vi "multi-function-fpga3.vi"() -> ()   [LabVIEW 2016]
uses:
  <vilib>/rvi/Emulation/niFpgaGetClockAttributes.vi
  <vilib>/rvi/Emulation/niFpgaSctlEmulationGetInTimedLoop.vi
  <vilib>/rvi/Emulation/niFpgaEmulationReportErrorSimple.vi
  <vilib>/rvi/eio/common/nirviEmuTemplateMethod_errors.vi
  <vilib>/rvi/Emulation/niFpgaCriticalErrorInLSC.vi
  <vilib>/eio/EIONode/EIONode.xnode
panel:
  in  "Reset buttons":T1
  in  "Channel15":T2={"Ctrl"=enum."OFF", "scan end"=3.5, "scan begin"=0.0, "scan step"=0.0, "main input"=enum."DIO0", "sub input"=enum."DIO0", "boolean low"=3.5, "boolean high"=0.0} {"boolean high" format="%#_17g"; "boolean low" format="%#_17g"; "scan step" format="%#_17g"; "scan begin" format="%#_17g"; "scan end" format="%#_17g"}
  in  "Channel14":T2={"Ctrl"=enum."OFF", "scan end"=3.5, "scan begin"=0.0, "scan step"=0.0, "main input"=enum."DIO0", "sub input"=enum."DIO0", "boolean low"=3.5, "boolean high"=0.0} {"boolean high" format="%#_17g"; "boolean low" format="%#_17g"; "scan step" format="%#_17g"; "scan begin" format="%#_17g"; "scan end" format="%#_17g"}
  in  "Channel13":T2={"Ctrl"=enum."OFF", "scan end"=3.5, "scan begin"=0.0, "scan step"=0.0, "main input"=enum."DIO0", "sub input"=enum."DIO0", "boolean low"=3.5, "boolean high"=0.0} {"boolean high" format="%#_17g"; "boolean low" format="%#_17g"; "scan step" format="%#_17g"; "scan begin" format="%#_17g"; "scan end" format="%#_17g"}
  in  "Channel12":T2={"Ctrl"=enum."OFF", "scan end"=3.5, "scan begin"=0.0, "scan step"=0.0, "main input"=enum."DIO0", "sub input"=enum."DIO0", "boolean low"=3.5, "boolean high"=0.0} {"boolean high" format="%#_17g"; "boolean low" format="%#_17g"; "scan step" format="%#_17g"; "scan begin" format="%#_17g"; "scan end" format="%#_17g"}
  in  "Channel11":T2={"Ctrl"=enum."OFF", "scan end"=3.5, "scan begin"=0.0, "scan step"=0.0, "main input"=enum."DIO0", "sub input"=enum."DIO0", "boolean low"=3.5, "boolean high"=0.0} {"boolean high" format="%#_17g"; "boolean low" format="%#_17g"; "scan step" format="%#_17g"; "scan begin" format="%#_17g"; "scan end" format="%#_17g"}
  in  "Channel10":T2={"Ctrl"=enum."OFF", "scan end"=3.5, "scan begin"=0.0, "scan step"=0.0, "main input"=enum."DIO0", "sub input"=enum."DIO0", "boolean low"=3.5, "boolean high"=0.0} {"boolean high" format="%#_17g"; "boolean low" format="%#_17g"; "scan step" format="%#_17g"; "scan begin" format="%#_17g"; "scan end" format="%#_17g"}
  in  "Channel9":T2={"Ctrl"=enum."OFF", "scan end"=3.5, "scan begin"=0.0, "scan step"=0.0, "main input"=enum."DIO0", "sub input"=enum."DIO0", "boolean low"=3.5, "boolean high"=0.0} {"boolean high" format="%#_17g"; "boolean low" format="%#_17g"; "scan step" format="%#_17g"; "scan begin" format="%#_17g"; "scan end" format="%#_17g"}
  in  "Channel8":T2={"Ctrl"=enum."OFF", "scan end"=3.5, "scan begin"=0.0, "scan step"=0.0, "main input"=enum."DIO0", "sub input"=enum."DIO0", "boolean low"=3.5, "boolean high"=0.0} {"boolean high" format="%#_17g"; "boolean low" format="%#_17g"; "scan step" format="%#_17g"; "scan begin" format="%#_17g"; "scan end" format="%#_17g"}
  in  "Channel7":T2={"Ctrl"=enum."OFF", "scan end"=3.5, "scan begin"=0.0, "scan step"=0.0, "main input"=enum."DIO0", "sub input"=enum."DIO0", "boolean low"=3.5, "boolean high"=0.0} {"boolean high" format="%#_17g"; "boolean low" format="%#_17g"; "scan step" format="%#_17g"; "scan begin" format="%#_17g"; "scan end" format="%#_17g"}
  in  "Channel6":T2={"Ctrl"=enum."OFF", "scan end"=3.5, "scan begin"=0.0, "scan step"=0.0, "main input"=enum."DIO0", "sub input"=enum."DIO0", "boolean low"=3.5, "boolean high"=0.0} {"boolean high" format="%#_17g"; "boolean low" format="%#_17g"; "scan step" format="%#_17g"; "scan begin" format="%#_17g"; "scan end" format="%#_17g"}
  in  "Channel5":T2={"Ctrl"=enum."OFF", "scan end"=3.5, "scan begin"=0.0, "scan step"=0.0, "main input"=enum."DIO0", "sub input"=enum."DIO0", "boolean low"=3.5, "boolean high"=0.0} {"boolean high" format="%#_17g"; "boolean low" format="%#_17g"; "scan step" format="%#_17g"; "scan begin" format="%#_17g"; "scan end" format="%#_17g"}
  in  "Channel4":T2={"Ctrl"=enum."OFF", "scan end"=3.5, "scan begin"=0.0, "scan step"=0.0, "main input"=enum."DIO0", "sub input"=enum."DIO0", "boolean low"=3.5, "boolean high"=0.0} {"boolean high" format="%#_17g"; "boolean low" format="%#_17g"; "scan step" format="%#_17g"; "scan begin" format="%#_17g"; "scan end" format="%#_17g"}
  in  "Channel3":T2={"Ctrl"=enum."OFF", "scan end"=3.5, "scan begin"=0.0, "scan step"=0.0, "main input"=enum."DIO0", "sub input"=enum."DIO0", "boolean low"=3.5, "boolean high"=0.0} {"boolean high" format="%#_17g"; "boolean low" format="%#_17g"; "scan step" format="%#_17g"; "scan begin" format="%#_17g"; "scan end" format="%#_17g"}
  in  "Channel2":T2={"Ctrl"=enum."OFF", "scan end"=3.5, "scan begin"=0.0, "scan step"=0.0, "main input"=enum."DIO0", "sub input"=enum."DIO0", "boolean low"=3.5, "boolean high"=0.0} {"boolean high" format="%#_17g"; "boolean low" format="%#_17g"; "scan step" format="%#_17g"; "scan begin" format="%#_17g"; "scan end" format="%#_17g"}
  in  "Channel1":T2={"Ctrl"=enum."OFF", "scan end"=3.5, "scan begin"=0.0, "scan step"=0.0, "main input"=enum."DIO0", "sub input"=enum."DIO0", "boolean low"=3.5, "boolean high"=0.0} {"boolean high" format="%#_17g"; "boolean low" format="%#_17g"; "scan step" format="%#_17g"; "scan begin" format="%#_17g"; "scan end" format="%#_17g"}
  in  "Channel0":T2={"Ctrl"=enum."OFF", "scan end"=3.5, "scan begin"=0.0, "scan step"=0.0, "main input"=enum."DIO0", "sub input"=enum."DIO0", "boolean low"=3.5, "boolean high"=0.0} {"boolean high" format="%#_17g"; "boolean low" format="%#_17g"; "scan step" format="%#_17g"; "scan begin" format="%#_17g"; "scan end" format="%#_17g"}
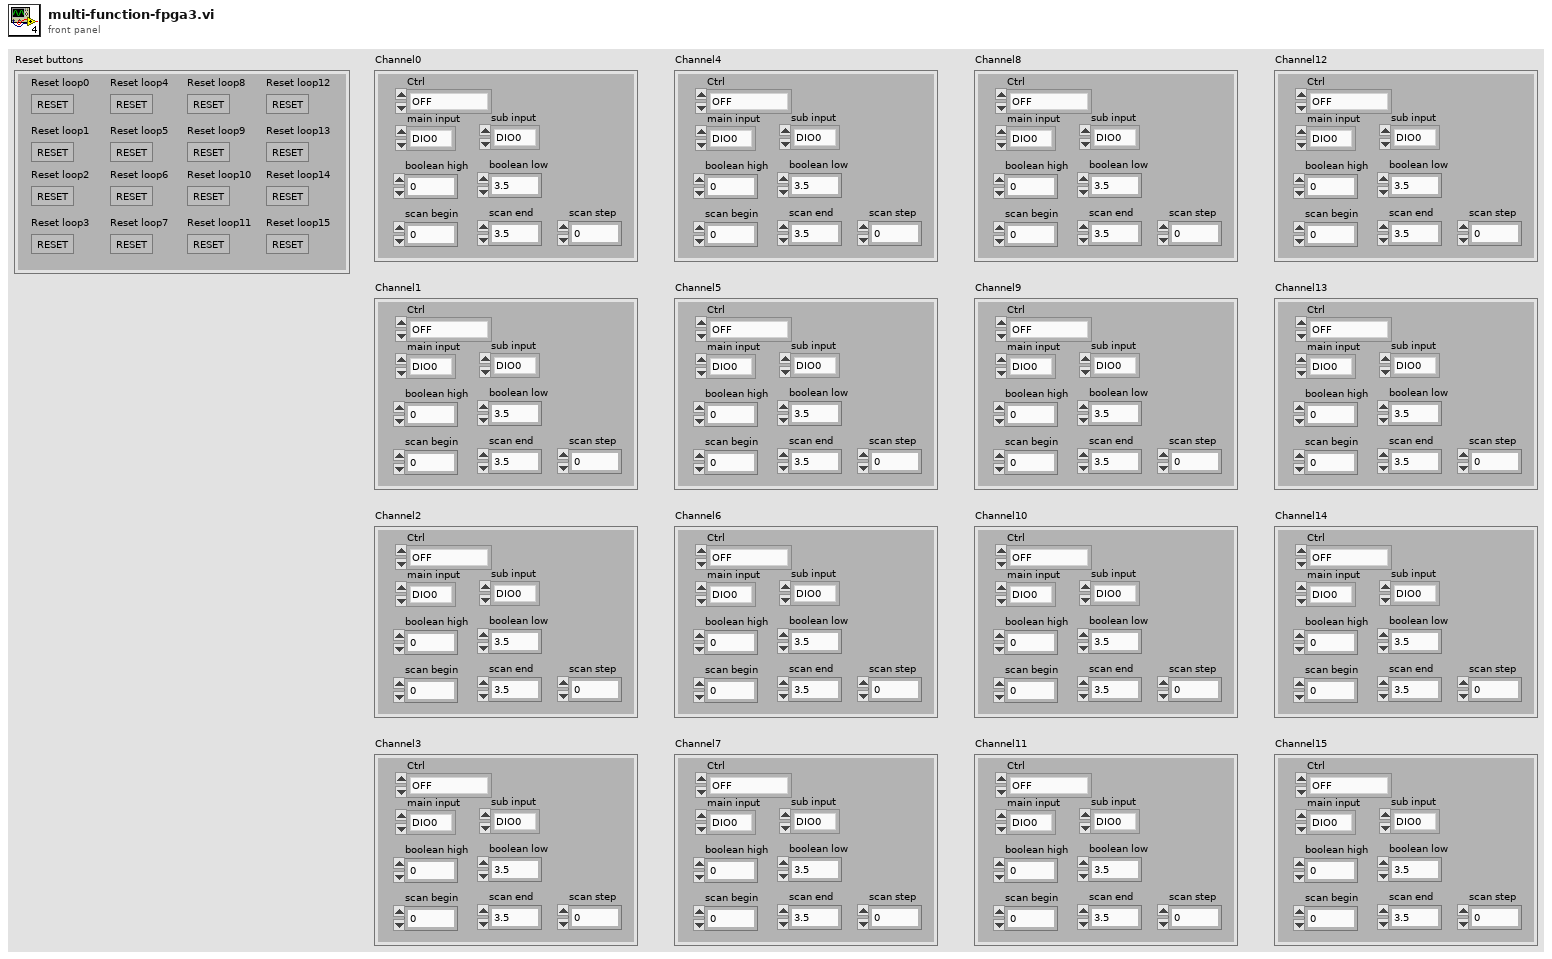
[diagram p1: front panel]
types:
  T1 = cluster{"Reset loop0":bool, "Reset loop1":bool, "Reset loop2":bool, "Reset loop3":bool, "Reset loop4":bool, "Reset loop5":bool, "Reset loop6":bool, "Reset loop7":bool, "Reset loop8":bool, "Reset loop9":bool, "Reset loop10":bool, "Reset loop11":bool, "Reset loop12":bool, "Reset loop13":bool, "Reset loop14":bool, "Reset loop15":bool}
  T2 = cluster{"Ctrl":enum16{"OFF", "SWITCH", "AND GATE", "OR GATE", "ITERATION"}, "scan end":sgl, "scan begin":sgl, "scan step":sgl, "main input":enum16{"DIO0", "DIO1", "DIO2", "DIO3", "DIO4", "DIO5", "DIO6", "DIO7", "DIO8", "DIO9", "DIO10", "DIO11", "DIO12", "DIO13", "DIO14", "DIO15", "DIO16", "DIO17", "DIO18", "DIO19", "DIO20", "DIO21", "DIO22", "DIO23", "DIO24", "DIO25", "DIO26", "DIO27", "DIO28", "DIO29", "DIO30", "DIO31"}, "sub input":enum16{"DIO0", "DIO1", "DIO2", "DIO3", "DIO4", "DIO5", "DIO6", "DIO7", "DIO8", "DIO9", "DIO10", "DIO11", "DIO12", "DIO13", "DIO14", "DIO15", "DIO16", "DIO17", "DIO18", "DIO19", "DIO20", "DIO21", "DIO22", "DIO23", "DIO24", "DIO25", "DIO26", "DIO27", "DIO28", "DIO29", "DIO30", "DIO31"}, "boolean low":sgl, "boolean high":sgl}
  T3 = enum16{"OFF", "SWITCH", "AND GATE", "OR GATE", "ITERATION"}
  T4 = enum16{"DIO0", "DIO1", "DIO2", "DIO3", "DIO4", "DIO5", "DIO6", "DIO7", "DIO8", "DIO9", "DIO10", "DIO11", "DIO12", "DIO13", "DIO14", "DIO15", "DIO16", "DIO17", "DIO18", "DIO19", "DIO20", "DIO21", "DIO22", "DIO23", "DIO24", "DIO25", "DIO26", "DIO27", "DIO28", "DIO29", "DIO30", "DIO31"}
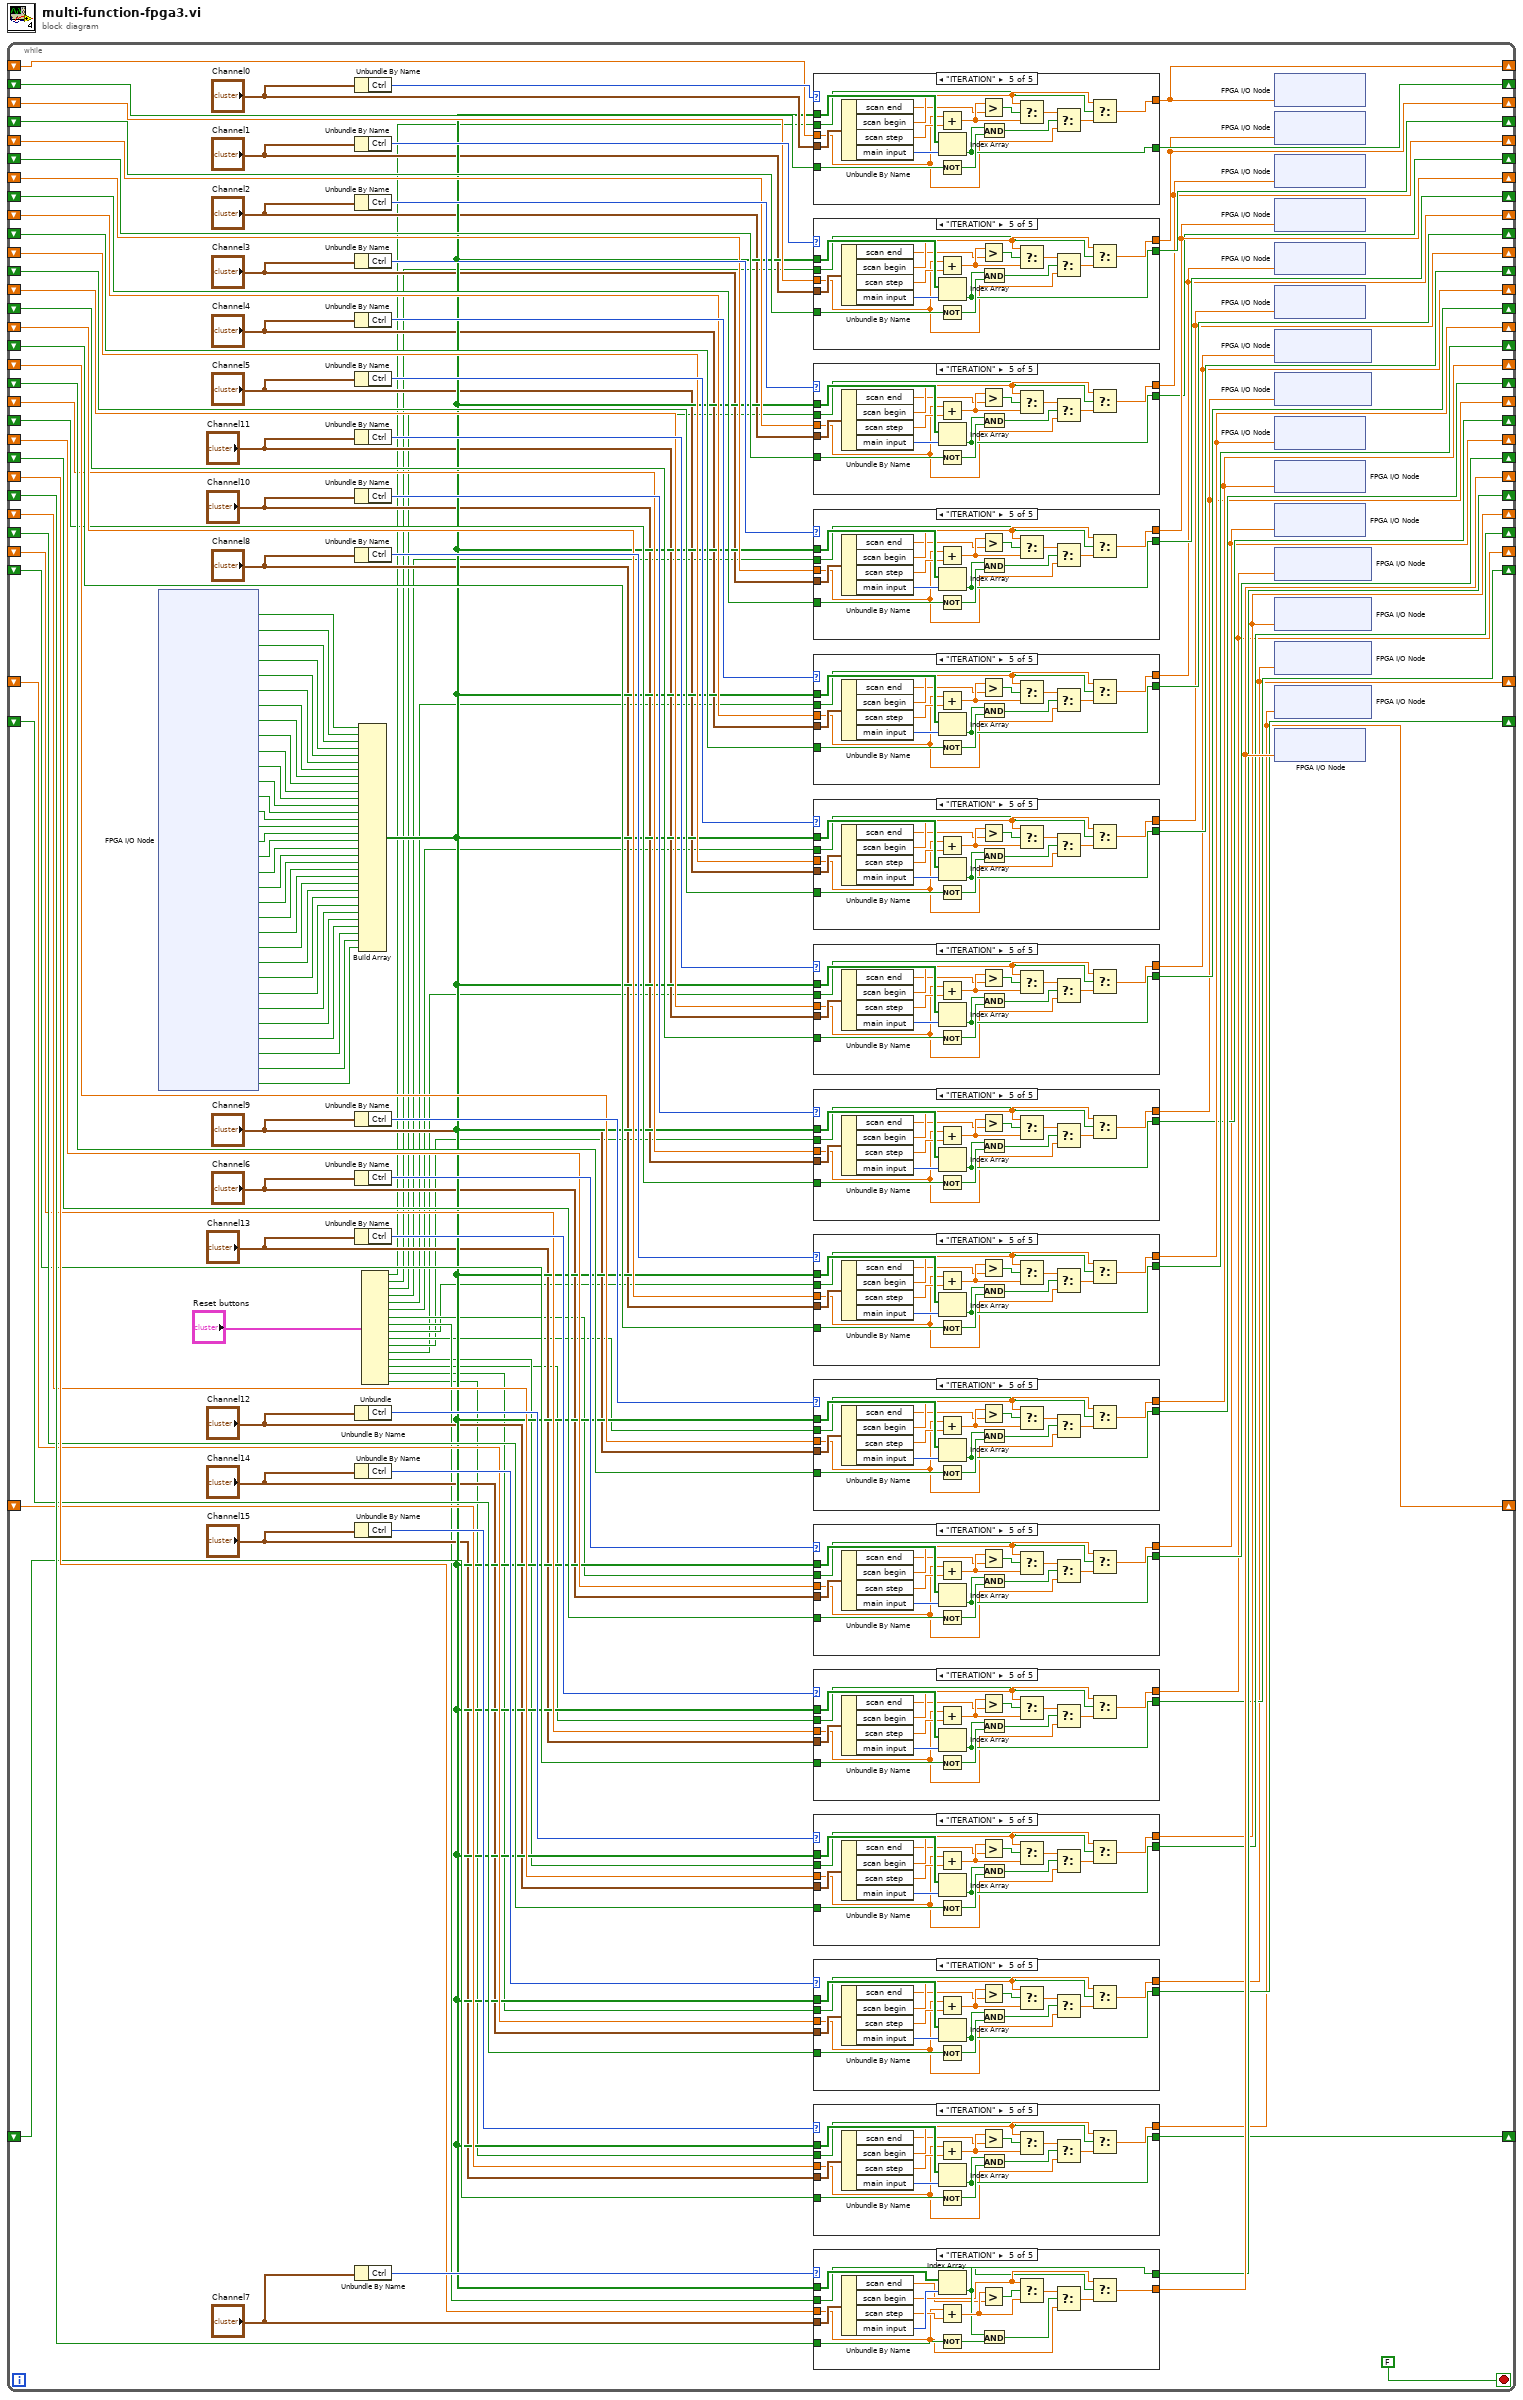
[diagram p0: block diagram]
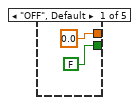
[diagram p2: hidden frame]
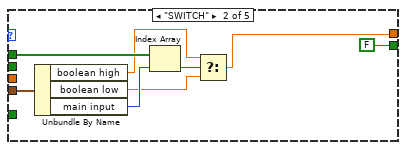
[diagram p3: hidden frame]
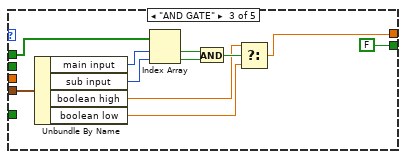
[diagram p4: hidden frame]
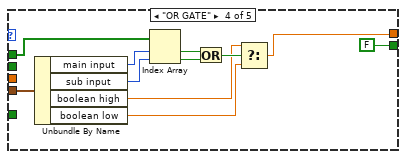
[diagram p5: hidden frame]
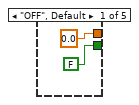
[diagram p6: hidden frame]
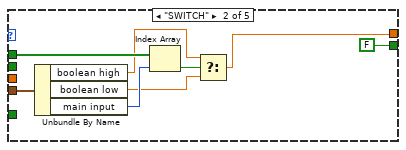
[diagram p7: hidden frame]
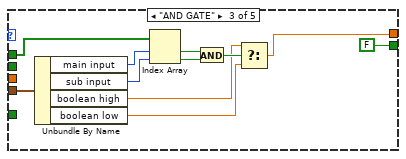
[diagram p8: hidden frame]
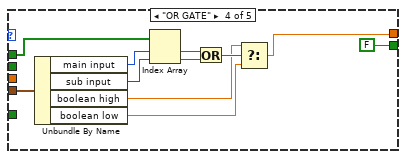
[diagram p9: hidden frame]
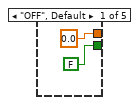
[diagram p10: hidden frame]
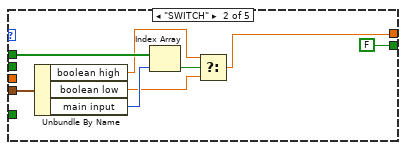
[diagram p11: hidden frame]
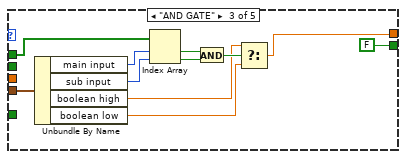
[diagram p12: hidden frame]
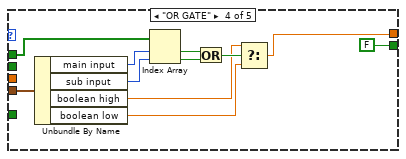
[diagram p13: hidden frame]
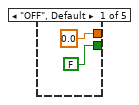
[diagram p14: hidden frame]
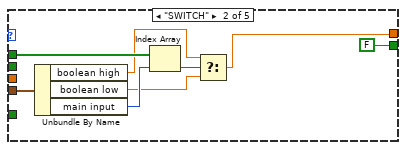
[diagram p15: hidden frame]
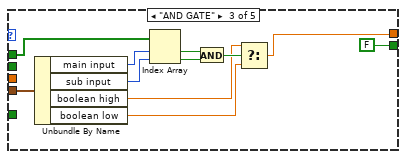
[diagram p16: hidden frame]
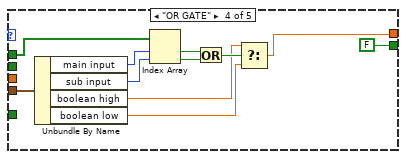
[diagram p17: hidden frame]
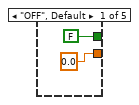
[diagram p18: hidden frame]
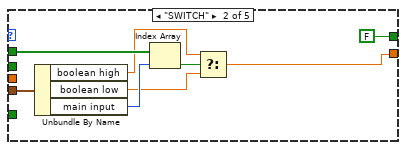
[diagram p19: hidden frame]
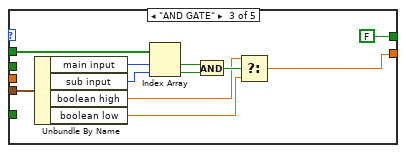
[diagram p20: hidden frame]
diagram:
  n1 = while {
    shift-right: [w113] -> _
    shift-left: _ -> [w111]
    shift-right: [w110] -> _
    shift-left: _ -> [w109]
    shift-right: [w107] -> _
    shift-left: _ -> [w105]
    shift-right: [w106] -> _
    shift-left: _ -> [w104]
    shift-right: [w99] -> _
    shift-left: _ -> [w97]
    shift-right: [w98] -> _
    shift-left: _ -> [w96]
    shift-right: [w101] -> _
    shift-left: _ -> [w95]
    shift-right: [w100] -> _
    shift-left: _ -> [w94]
    shift-right: [w89] -> _
    shift-left: _ -> [w81]
    shift-right: [w88] -> _
    shift-left: _ -> [w80]
    shift-right: [w87] -> _
    shift-left: _ -> [w79]
    shift-right: [w86] -> _
    shift-left: _ -> [w78]
    shift-right: [w85] -> _
    shift-left: _ -> [w77]
    shift-right: [w84] -> _
    shift-left: _ -> [w76]
    shift-right: [w83] -> _
    shift-left: _ -> [w75]
    shift-right: [w82] -> _
    shift-left: _ -> [w74]
    shift-right: [w65] -> _
    shift-left: _ -> [w49]
    shift-right: [w64] -> _
    shift-left: _ -> [w48]
    shift-right: [w63] -> _
    shift-left: _ -> [w47]
    shift-right: [w62] -> _
    shift-left: _ -> [w46]
    shift-right: [w61] -> _
    shift-left: _ -> [w45]
    shift-right: [w60] -> _
    shift-left: _ -> [w44]
    shift-right: [w59] -> _
    shift-left: _ -> [w43]
    shift-right: [w58] -> _
    shift-left: _ -> [w42]
    shift-right: [w57] -> _
    shift-left: _ -> [w41]
    shift-right: [w56] -> _
    shift-left: _ -> [w40]
    shift-right: [w55] -> _
    shift-left: _ -> [w39]
    shift-right: [w54] -> _
    shift-left: _ -> [w38]
    shift-right: [w53] -> _
    shift-left: _ -> [w37]
    shift-right: [w52] -> _
    shift-left: _ -> [w36]
    shift-right: [w51] -> _
    shift-left: _ -> [w35]
    shift-right: [w50] -> _
    shift-left: _ -> [w34]
    stop <- FALSE stop-if-true
    n2 = xnode "FPGA I/O Node"() -> ("Mod2/DIO0"=w146:bool, "Mod2/DIO1"=w145:bool, "Mod2/DIO2"=w144:bool, "Mod2/DIO3"=w143:bool, "Mod2/DIO4"=w142:bool, "Mod2/DIO5"=w141:bool, "Mod2/DIO6"=w140:bool, "Mod2/DIO7"=w139:bool, "Mod2/DIO8"=w138:bool, "Mod2/DIO9"=w137:bool, "Mod2/DIO10"=w136:bool, "Mod2/DIO11"=w135:bool, "Mod2/DIO12"=w134:bool, "Mod2/DIO13"=w133:bool, "Mod2/DIO14"=w132:bool, "Mod2/DIO15"=w131:bool, "Mod2/DIO16"=w130:bool, "Mod2/DIO17"=w129:bool, "Mod2/DIO18"=w128:bool, "Mod2/DIO19"=w127:bool, "Mod2/DIO20"=w126:bool, "Mod2/DIO21"=w125:bool, "Mod2/DIO22"=w124:bool, "Mod2/DIO23"=w123:bool, "Mod2/DIO24"=w122:bool, "Mod2/DIO25"=w121:bool, "Mod2/DIO26"=w120:bool, "Mod2/DIO27"=w119:bool, "Mod2/DIO28"=w118:bool, "Mod2/DIO29"=w117:bool, "Mod2/DIO30"=w116:bool, "Mod2/DIO31"=w115:bool)  [unwired: 32 in, 32 out]
    n3 = Unbundle By Name("Channel0") -> ("Ctrl"=w114:T3)
    n4 = Unbundle By Name("Channel1") -> ("Ctrl"=w108:T3)
    n5 = Unbundle By Name("Channel2") -> ("Ctrl"=w103:T3)
    n6 = Unbundle By Name("Channel3") -> ("Ctrl"=w102:T3)
    n7 = Unbundle By Name("Channel4") -> ("Ctrl"=w93:T3)
    n8 = Unbundle By Name("Channel5") -> ("Ctrl"=w92:T3)
    n9 = Unbundle By Name("Channel11") -> ("Ctrl"=w91:T3)
    n10 = Unbundle By Name("Channel10") -> ("Ctrl"=w72:T3)
    n11 = Unbundle By Name("Channel8") -> ("Ctrl"=w90:T3)
    n12 = Unbundle By Name("Channel9") -> ("Ctrl"=w73:T3)
    n13 = Unbundle By Name("Channel6") -> ("Ctrl"=w71:T3)
    n14 = Unbundle By Name("Channel13") -> ("Ctrl"=w68:T3)
    n15 = Unbundle By Name("Channel12") -> ("Ctrl"=w69:T3)
    n16 = Unbundle By Name("Channel14") -> ("Ctrl"=w67:T3)
    n17 = Unbundle By Name("Channel15") -> ("Ctrl"=w66:T3)
    n18 = Unbundle By Name("Channel7") -> ("Ctrl"=w70:T3)
    n19 = Build Array(w146, w145, w144, w143, w142, w141, w140, w139, w138, w137, w136, w135, w134, w133, w132, w131, w130, w129, w128, w127, w126, w125, w124, w123, w122, w121, w120, w119, w118, w117, w116, w115) -> (w33:bool[])
    n20 = Unbundle("Reset buttons") -> ("Reset loop0"=w16:bool, "Reset loop1"=w15:bool, "Reset loop2"=w14:bool, "Reset loop3"=w13:bool, "Reset loop4"=w12:bool, "Reset loop5"=w11:bool, "Reset loop6"=w10:bool, "Reset loop7"=w9:bool, "Reset loop8"=w8:bool, "Reset loop9"=w7:bool, "Reset loop10"=w6:bool, "Reset loop11"=w5:bool, "Reset loop12"=w4:bool, "Reset loop13"=w3:bool, "Reset loop14"=w2:bool, "Reset loop15"=w1:bool)
    n21 = case shown="\"ITERATION\"" w114 {
      tunnel: [sgl 0.0 w885 w894 w905 w916] -> w113
      tunnel: w33 -> [_ w892 w902 w906 w930]
      tunnel: "Channel0" -> [_ w891 w903 w907 w931]
      tunnel: w111 -> [_ _ _ _ w921]
      tunnel: [FALSE ("Mod2/DIO31") FALSE ("Mod2/DIO31") FALSE ("Mod2/DIO31") FALSE ("Mod2/DIO31") w923] -> w110
      tunnel: w109 -> [_ _ _ _ w925]
      tunnel: w16 -> [_ _ _ _ w915]
      frame "OFF", Default {
      }
      frame "SWITCH" {
        n22 = Unbundle By Name(w891) -> ("boolean high"=w887:sgl, "boolean low"=w888:sgl, "main input"=w890:T4)
        n23 = Index Array(array=w892, index=w890) -> (element=w889:bool)
        n24 = Select(t=w887, s=w889, f=w888) -> (s? t:f=w885:sgl)
      }
      frame "AND GATE" {
        n25 = Unbundle By Name(w903) -> ("main input"=w901:T4, "sub input"=w900:T4, "boolean high"=w896:sgl, "boolean low"=w895:sgl)
        n26 = Index Array(array=w902, index #1=w901, index #2=w900) -> (element #1=w899:bool, element #2=w898:bool)
        n27 = And(x=w899, y=w898) -> (x .and. y?=w897:bool)
        n28 = Select(t=w896, s=w897, f=w895) -> (s? t:f=w894:sgl)
      }
      frame "OR GATE" {
        n29 = Unbundle By Name(w907) -> ("main input"=w914:T4, "sub input"=w913:T4, "boolean high"=w909:sgl, "boolean low"=w908:sgl)
        n30 = Index Array(array=w906, index #1=w914, index #2=w913) -> (element #1=w912:bool, element #2=w911:bool)
        n31 = Or(x=w912, y=w911) -> (x .or. y?=w910:bool)
        n32 = Select(t=w909, s=w910, f=w908) -> (s? t:f=w905:sgl)
      }
      frame "ITERATION" {
        n33 = Unbundle By Name(w931) -> ("scan end"=w918:sgl, "scan begin"=w919:sgl, "scan step"=w928:sgl, "main input"=w929:T4)
        n34 = Add(x=w921, y=w928) -> (x+y=w926:sgl)
        n35 = Not(x=w925) -> (.not. x?=w924:bool)
        n36 = Index Array(array=w930, index=w929) -> (element=w923:bool)
        n37 = Greater?(x=w926, y=w918) -> (0:w927:bool)
        n38 = And(x=w923, y=w924) -> (x .and. y?=w922:bool)
        n39 = Select(t=w919, s=w927, f=w926) -> (s? t:f=w920:sgl)
        n40 = Select(t=w920, s=w922, f=w921) -> (s? t:f=w917:sgl)
        n41 = Select(t=w919, s=w915, f=w917) -> (s? t:f=w916:sgl)
      }
    }
    n42 = case shown="\"ITERATION\"" w108 {
      tunnel: [sgl 0.0 w836 w845 w856 w867] -> w107
      tunnel: w33 -> [_ w843 w853 w857 w881]
      tunnel: "Channel1" -> [_ w842 w854 w858 w882]
      tunnel: w105 -> [_ _ _ _ w872]
      tunnel: [FALSE ("Mod2/DIO31") FALSE ("Mod2/DIO31") FALSE ("Mod2/DIO31") FALSE ("Mod2/DIO31") w874] -> w106
      tunnel: w104 -> [_ _ _ _ w876]
      tunnel: w15 -> [_ _ _ _ w866]
      frame "OFF", Default {
      }
      frame "SWITCH" {
        n43 = Unbundle By Name(w842) -> ("boolean high"=w838:sgl, "boolean low"=w839:sgl, "main input"=w841:T4)
        n44 = Index Array(array=w843, index=w841) -> (element=w840:bool)
        n45 = Select(t=w838, s=w840, f=w839) -> (s? t:f=w836:sgl)
      }
      frame "AND GATE" {
        n46 = Unbundle By Name(w854) -> ("main input"=w852:T4, "sub input"=w851:T4, "boolean high"=w847:sgl, "boolean low"=w846:sgl)
        n47 = Index Array(array=w853, index #1=w852, index #2=w851) -> (element #1=w850:bool, element #2=w849:bool)
        n48 = And(x=w850, y=w849) -> (x .and. y?=w848:bool)
        n49 = Select(t=w847, s=w848, f=w846) -> (s? t:f=w845:sgl)
      }
      frame "OR GATE" {
        n50 = Unbundle By Name(w858) -> ("main input"=w865:T4, "sub input"=w864:T4, "boolean high"=w860:sgl, "boolean low"=w859:sgl)
        n51 = Index Array(array=w857, index #1=w865, index #2=w864) -> (element #1=w863:bool, element #2=w862:bool)
        n52 = Or(x=w863, y=w862) -> (x .or. y?=w861:bool)
        n53 = Select(t=w860, s=w861, f=w859) -> (s? t:f=w856:sgl)
      }
      frame "ITERATION" {
        n54 = Unbundle By Name(w882) -> ("scan end"=w869:sgl, "scan begin"=w870:sgl, "scan step"=w879:sgl, "main input"=w880:T4)
        n55 = Add(x=w872, y=w879) -> (x+y=w877:sgl)
        n56 = Not(x=w876) -> (.not. x?=w875:bool)
        n57 = Index Array(array=w881, index=w880) -> (element=w874:bool)
        n58 = Greater?(x=w877, y=w869) -> (0:w878:bool)
        n59 = And(x=w874, y=w875) -> (x .and. y?=w873:bool)
        n60 = Select(t=w870, s=w878, f=w877) -> (s? t:f=w871:sgl)
        n61 = Select(t=w871, s=w873, f=w872) -> (s? t:f=w868:sgl)
        n62 = Select(t=w870, s=w866, f=w868) -> (s? t:f=w867:sgl)
      }
    }
    n63 = case shown="\"ITERATION\"" w103 {
      tunnel: [sgl 0.0 w787 w796 w807 w818] -> w99
      tunnel: w33 -> [_ w794 w804 w808 w832]
      tunnel: "Channel2" -> [_ w793 w805 w809 w833]
      tunnel: w97 -> [_ _ _ _ w823]
      tunnel: [FALSE ("Mod2/DIO31") FALSE ("Mod2/DIO31") FALSE ("Mod2/DIO31") FALSE ("Mod2/DIO31") w825] -> w98
      tunnel: w96 -> [_ _ _ _ w827]
      tunnel: w14 -> [_ _ _ _ w817]
      frame "OFF", Default {
      }
      frame "SWITCH" {
        n64 = Unbundle By Name(w793) -> ("boolean high"=w789:sgl, "boolean low"=w790:sgl, "main input"=w792:T4)
        n65 = Index Array(array=w794, index=w792) -> (element=w791:bool)
        n66 = Select(t=w789, s=w791, f=w790) -> (s? t:f=w787:sgl)
      }
      frame "AND GATE" {
        n67 = Unbundle By Name(w805) -> ("main input"=w803:T4, "sub input"=w802:T4, "boolean high"=w798:sgl, "boolean low"=w797:sgl)
        n68 = Index Array(array=w804, index #1=w803, index #2=w802) -> (element #1=w801:bool, element #2=w800:bool)
        n69 = And(x=w801, y=w800) -> (x .and. y?=w799:bool)
        n70 = Select(t=w798, s=w799, f=w797) -> (s? t:f=w796:sgl)
      }
      frame "OR GATE" {
        n71 = Unbundle By Name(w809) -> ("main input"=w816:T4, "sub input"=w815:T4, "boolean high"=w811:sgl, "boolean low"=w810:sgl)
        n72 = Index Array(array=w808, index #1=w816, index #2=w815) -> (element #1=w814:bool, element #2=w813:bool)
        n73 = Or(x=w814, y=w813) -> (x .or. y?=w812:bool)
        n74 = Select(t=w811, s=w812, f=w810) -> (s? t:f=w807:sgl)
      }
      frame "ITERATION" {
        n75 = Unbundle By Name(w833) -> ("scan end"=w820:sgl, "scan begin"=w821:sgl, "scan step"=w830:sgl, "main input"=w831:T4)
        n76 = Add(x=w823, y=w830) -> (x+y=w828:sgl)
        n77 = Not(x=w827) -> (.not. x?=w826:bool)
        n78 = Index Array(array=w832, index=w831) -> (element=w825:bool)
        n79 = Greater?(x=w828, y=w820) -> (0:w829:bool)
        n80 = And(x=w825, y=w826) -> (x .and. y?=w824:bool)
        n81 = Select(t=w821, s=w829, f=w828) -> (s? t:f=w822:sgl)
        n82 = Select(t=w822, s=w824, f=w823) -> (s? t:f=w819:sgl)
        n83 = Select(t=w821, s=w817, f=w819) -> (s? t:f=w818:sgl)
      }
    }
    n84 = case shown="\"ITERATION\"" w102 {
      tunnel: [sgl 0.0 w738 w747 w758 w769] -> w101
      tunnel: w33 -> [_ w745 w755 w759 w783]
      tunnel: "Channel3" -> [_ w744 w756 w760 w784]
      tunnel: w95 -> [_ _ _ _ w774]
      tunnel: [FALSE ("Mod2/DIO31") FALSE ("Mod2/DIO31") FALSE ("Mod2/DIO31") FALSE ("Mod2/DIO31") w776] -> w100
      tunnel: w94 -> [_ _ _ _ w778]
      tunnel: w13 -> [_ _ _ _ w768]
      frame "OFF", Default {
      }
      frame "SWITCH" {
        n85 = Unbundle By Name(w744) -> ("boolean high"=w740:sgl, "boolean low"=w741:sgl, "main input"=w743:T4)
        n86 = Index Array(array=w745, index=w743) -> (element=w742:bool)
        n87 = Select(t=w740, s=w742, f=w741) -> (s? t:f=w738:sgl)
      }
      frame "AND GATE" {
        n88 = Unbundle By Name(w756) -> ("main input"=w754:T4, "sub input"=w753:T4, "boolean high"=w749:sgl, "boolean low"=w748:sgl)
        n89 = Index Array(array=w755, index #1=w754, index #2=w753) -> (element #1=w752:bool, element #2=w751:bool)
        n90 = And(x=w752, y=w751) -> (x .and. y?=w750:bool)
        n91 = Select(t=w749, s=w750, f=w748) -> (s? t:f=w747:sgl)
      }
      frame "OR GATE" {
        n92 = Unbundle By Name(w760) -> ("main input"=w767:T4, "sub input"=w766:T4, "boolean high"=w762:sgl, "boolean low"=w761:sgl)
        n93 = Index Array(array=w759, index #1=w767, index #2=w766) -> (element #1=w765:bool, element #2=w764:bool)
        n94 = Or(x=w765, y=w764) -> (x .or. y?=w763:bool)
        n95 = Select(t=w762, s=w763, f=w761) -> (s? t:f=w758:sgl)
      }
      frame "ITERATION" {
        n96 = Unbundle By Name(w784) -> ("scan end"=w771:sgl, "scan begin"=w772:sgl, "scan step"=w781:sgl, "main input"=w782:T4)
        n97 = Add(x=w774, y=w781) -> (x+y=w779:sgl)
        n98 = Not(x=w778) -> (.not. x?=w777:bool)
        n99 = Index Array(array=w783, index=w782) -> (element=w776:bool)
        n100 = Greater?(x=w779, y=w771) -> (0:w780:bool)
        n101 = And(x=w776, y=w777) -> (x .and. y?=w775:bool)
        n102 = Select(t=w772, s=w780, f=w779) -> (s? t:f=w773:sgl)
        n103 = Select(t=w773, s=w775, f=w774) -> (s? t:f=w770:sgl)
        n104 = Select(t=w772, s=w768, f=w770) -> (s? t:f=w769:sgl)
      }
    }
    n105 = case shown="\"ITERATION\"" w93 {
      tunnel: [sgl 0.0 w689 w698 w709 w720] -> w89
      tunnel: w33 -> [_ w696 w706 w710 w734]
      tunnel: "Channel4" -> [_ w695 w707 w711 w735]
      tunnel: w81 -> [_ _ _ _ w725]
      tunnel: [FALSE ("Mod2/DIO31") FALSE ("Mod2/DIO31") FALSE ("Mod2/DIO31") FALSE ("Mod2/DIO31") w727] -> w88
      tunnel: w80 -> [_ _ _ _ w729]
      tunnel: w12 -> [_ _ _ _ w719]
      frame "OFF", Default {
      }
      frame "SWITCH" {
        n106 = Unbundle By Name(w695) -> ("boolean high"=w691:sgl, "boolean low"=w692:sgl, "main input"=w694:T4)
        n107 = Index Array(array=w696, index=w694) -> (element=w693:bool)
        n108 = Select(t=w691, s=w693, f=w692) -> (s? t:f=w689:sgl)
      }
      frame "AND GATE" {
        n109 = Unbundle By Name(w707) -> ("main input"=w705:T4, "sub input"=w704:T4, "boolean high"=w700:sgl, "boolean low"=w699:sgl)
        n110 = Index Array(array=w706, index #1=w705, index #2=w704) -> (element #1=w703:bool, element #2=w702:bool)
        n111 = And(x=w703, y=w702) -> (x .and. y?=w701:bool)
        n112 = Select(t=w700, s=w701, f=w699) -> (s? t:f=w698:sgl)
      }
      frame "OR GATE" {
        n113 = Unbundle By Name(w711) -> ("main input"=w718:T4, "sub input"=w717:T4, "boolean high"=w713:sgl, "boolean low"=w712:sgl)
        n114 = Index Array(array=w710, index #1=w718, index #2=w717) -> (element #1=w716:bool, element #2=w715:bool)
        n115 = Or(x=w716, y=w715) -> (x .or. y?=w714:bool)
        n116 = Select(t=w713, s=w714, f=w712) -> (s? t:f=w709:sgl)
      }
      frame "ITERATION" {
        n117 = Unbundle By Name(w735) -> ("scan end"=w722:sgl, "scan begin"=w723:sgl, "scan step"=w732:sgl, "main input"=w733:T4)
        n118 = Add(x=w725, y=w732) -> (x+y=w730:sgl)
        n119 = Not(x=w729) -> (.not. x?=w728:bool)
        n120 = Index Array(array=w734, index=w733) -> (element=w727:bool)
        n121 = Greater?(x=w730, y=w722) -> (0:w731:bool)
        n122 = And(x=w727, y=w728) -> (x .and. y?=w726:bool)
        n123 = Select(t=w723, s=w731, f=w730) -> (s? t:f=w724:sgl)
        n124 = Select(t=w724, s=w726, f=w725) -> (s? t:f=w721:sgl)
        n125 = Select(t=w723, s=w719, f=w721) -> (s? t:f=w720:sgl)
      }
    }
    n126 = case shown="\"ITERATION\"" w92 {
      tunnel: [sgl 0.0 w640 w649 w660 w671] -> w87
      tunnel: w33 -> [_ w647 w657 w661 w685]
      tunnel: "Channel5" -> [_ w646 w658 w662 w686]
      tunnel: w79 -> [_ _ _ _ w676]
      tunnel: [FALSE ("Mod2/DIO31") FALSE ("Mod2/DIO31") FALSE ("Mod2/DIO31") FALSE ("Mod2/DIO31") w678] -> w86
      tunnel: w78 -> [_ _ _ _ w680]
      tunnel: w11 -> [_ _ _ _ w670]
      frame "OFF", Default {
      }
      frame "SWITCH" {
        n127 = Unbundle By Name(w646) -> ("boolean high"=w642:sgl, "boolean low"=w643:sgl, "main input"=w645:T4)
        n128 = Index Array(array=w647, index=w645) -> (element=w644:bool)
        n129 = Select(t=w642, s=w644, f=w643) -> (s? t:f=w640:sgl)
      }
      frame "AND GATE" {
        n130 = Unbundle By Name(w658) -> ("main input"=w656:T4, "sub input"=w655:T4, "boolean high"=w651:sgl, "boolean low"=w650:sgl)
        n131 = Index Array(array=w657, index #1=w656, index #2=w655) -> (element #1=w654:bool, element #2=w653:bool)
        n132 = And(x=w654, y=w653) -> (x .and. y?=w652:bool)
        n133 = Select(t=w651, s=w652, f=w650) -> (s? t:f=w649:sgl)
      }
      frame "OR GATE" {
        n134 = Unbundle By Name(w662) -> ("main input"=w669:T4, "sub input"=w668:T4, "boolean high"=w664:sgl, "boolean low"=w663:sgl)
        n135 = Index Array(array=w661, index #1=w669, index #2=w668) -> (element #1=w667:bool, element #2=w666:bool)
        n136 = Or(x=w667, y=w666) -> (x .or. y?=w665:bool)
        n137 = Select(t=w664, s=w665, f=w663) -> (s? t:f=w660:sgl)
      }
      frame "ITERATION" {
        n138 = Unbundle By Name(w686) -> ("scan end"=w673:sgl, "scan begin"=w674:sgl, "scan step"=w683:sgl, "main input"=w684:T4)
        n139 = Add(x=w676, y=w683) -> (x+y=w681:sgl)
        n140 = Not(x=w680) -> (.not. x?=w679:bool)
        n141 = Index Array(array=w685, index=w684) -> (element=w678:bool)
        n142 = Greater?(x=w681, y=w673) -> (0:w682:bool)
        n143 = And(x=w678, y=w679) -> (x .and. y?=w677:bool)
        n144 = Select(t=w674, s=w682, f=w681) -> (s? t:f=w675:sgl)
        n145 = Select(t=w675, s=w677, f=w676) -> (s? t:f=w672:sgl)
        n146 = Select(t=w674, s=w670, f=w672) -> (s? t:f=w671:sgl)
      }
    }
    n147 = case shown="\"ITERATION\"" w91 {
      tunnel: [sgl 0.0 w591 w600 w611 w622] -> w85
      tunnel: w33 -> [_ w598 w608 w612 w636]
      tunnel: "Channel11" -> [_ w597 w609 w613 w637]
      tunnel: w77 -> [_ _ _ _ w627]
      tunnel: [FALSE ("Mod2/DIO31") FALSE ("Mod2/DIO31") FALSE ("Mod2/DIO31") FALSE ("Mod2/DIO31") w629] -> w84
      tunnel: w76 -> [_ _ _ _ w631]
      tunnel: w5 -> [_ _ _ _ w621]
      frame "OFF", Default {
      }
      frame "SWITCH" {
        n148 = Unbundle By Name(w597) -> ("boolean high"=w593:sgl, "boolean low"=w594:sgl, "main input"=w596:T4)
        n149 = Index Array(array=w598, index=w596) -> (element=w595:bool)
        n150 = Select(t=w593, s=w595, f=w594) -> (s? t:f=w591:sgl)
      }
      frame "AND GATE" {
        n151 = Unbundle By Name(w609) -> ("main input"=w607:T4, "sub input"=w606:T4, "boolean high"=w602:sgl, "boolean low"=w601:sgl)
        n152 = Index Array(array=w608, index #1=w607, index #2=w606) -> (element #1=w605:bool, element #2=w604:bool)
        n153 = And(x=w605, y=w604) -> (x .and. y?=w603:bool)
        n154 = Select(t=w602, s=w603, f=w601) -> (s? t:f=w600:sgl)
      }
      frame "OR GATE" {
        n155 = Unbundle By Name(w613) -> ("main input"=w620:T4, "sub input"=w619:T4, "boolean high"=w615:sgl, "boolean low"=w614:sgl)
        n156 = Index Array(array=w612, index #1=w620, index #2=w619) -> (element #1=w618:bool, element #2=w617:bool)
        n157 = Or(x=w618, y=w617) -> (x .or. y?=w616:bool)
        n158 = Select(t=w615, s=w616, f=w614) -> (s? t:f=w611:sgl)
      }
      frame "ITERATION" {
        n159 = Unbundle By Name(w637) -> ("scan end"=w624:sgl, "scan begin"=w625:sgl, "scan step"=w634:sgl, "main input"=w635:T4)
        n160 = Add(x=w627, y=w634) -> (x+y=w632:sgl)
        n161 = Not(x=w631) -> (.not. x?=w630:bool)
        n162 = Index Array(array=w636, index=w635) -> (element=w629:bool)
        n163 = Greater?(x=w632, y=w624) -> (0:w633:bool)
        n164 = And(x=w629, y=w630) -> (x .and. y?=w628:bool)
        n165 = Select(t=w625, s=w633, f=w632) -> (s? t:f=w626:sgl)
        n166 = Select(t=w626, s=w628, f=w627) -> (s? t:f=w623:sgl)
        n167 = Select(t=w625, s=w621, f=w623) -> (s? t:f=w622:sgl)
      }
    }
    n168 = case shown="\"ITERATION\"" w72 {
      tunnel: [sgl 0.0 w444 w453 w464 w475] -> w63
      tunnel: w33 -> [_ w451 w461 w465 w489]
      tunnel: "Channel10" -> [_ w450 w462 w466 w490]
      tunnel: w47 -> [_ _ _ _ w480]
      tunnel: [FALSE ("Mod2/DIO31") FALSE ("Mod2/DIO31") FALSE ("Mod2/DIO31") FALSE ("Mod2/DIO31") w482] -> w62
      tunnel: w46 -> [_ _ _ _ w484]
      tunnel: w6 -> [_ _ _ _ w474]
      frame "OFF", Default {
      }
      frame "SWITCH" {
        n169 = Unbundle By Name(w450) -> ("boolean high"=w446:sgl, "boolean low"=w447:sgl, "main input"=w449:T4)
        n170 = Index Array(array=w451, index=w449) -> (element=w448:bool)
        n171 = Select(t=w446, s=w448, f=w447) -> (s? t:f=w444:sgl)
      }
      frame "AND GATE" {
        n172 = Unbundle By Name(w462) -> ("main input"=w460:T4, "sub input"=w459:T4, "boolean high"=w455:sgl, "boolean low"=w454:sgl)
        n173 = Index Array(array=w461, index #1=w460, index #2=w459) -> (element #1=w458:bool, element #2=w457:bool)
        n174 = And(x=w458, y=w457) -> (x .and. y?=w456:bool)
        n175 = Select(t=w455, s=w456, f=w454) -> (s? t:f=w453:sgl)
      }
      frame "OR GATE" {
        n176 = Unbundle By Name(w466) -> ("main input"=w473:T4, "sub input"=w472:T4, "boolean high"=w468:sgl, "boolean low"=w467:sgl)
        n177 = Index Array(array=w465, index #1=w473, index #2=w472) -> (element #1=w471:bool, element #2=w470:bool)
        n178 = Or(x=w471, y=w470) -> (x .or. y?=w469:bool)
        n179 = Select(t=w468, s=w469, f=w467) -> (s? t:f=w464:sgl)
      }
      frame "ITERATION" {
        n180 = Unbundle By Name(w490) -> ("scan end"=w477:sgl, "scan begin"=w478:sgl, "scan step"=w487:sgl, "main input"=w488:T4)
        n181 = Add(x=w480, y=w487) -> (x+y=w485:sgl)
        n182 = Not(x=w484) -> (.not. x?=w483:bool)
        n183 = Index Array(array=w489, index=w488) -> (element=w482:bool)
        n184 = Greater?(x=w485, y=w477) -> (0:w486:bool)
        n185 = And(x=w482, y=w483) -> (x .and. y?=w481:bool)
        n186 = Select(t=w478, s=w486, f=w485) -> (s? t:f=w479:sgl)
        n187 = Select(t=w479, s=w481, f=w480) -> (s? t:f=w476:sgl)
        n188 = Select(t=w478, s=w474, f=w476) -> (s? t:f=w475:sgl)
      }
    }
    n189 = case shown="\"ITERATION\"" w90 {
      tunnel: [sgl 0.0 w542 w551 w562 w573] -> w83
      tunnel: w33 -> [_ w549 w559 w563 w587]
      tunnel: "Channel8" -> [_ w548 w560 w564 w588]
      tunnel: w75 -> [_ _ _ _ w578]
      tunnel: [FALSE ("Mod2/DIO31") FALSE ("Mod2/DIO31") FALSE ("Mod2/DIO31") FALSE ("Mod2/DIO31") w580] -> w82
      tunnel: w74 -> [_ _ _ _ w582]
      tunnel: w8 -> [_ _ _ _ w572]
      frame "OFF", Default {
      }
      frame "SWITCH" {
        n190 = Unbundle By Name(w548) -> ("boolean high"=w544:sgl, "boolean low"=w545:sgl, "main input"=w547:T4)
        n191 = Index Array(array=w549, index=w547) -> (element=w546:bool)
        n192 = Select(t=w544, s=w546, f=w545) -> (s? t:f=w542:sgl)
      }
      frame "AND GATE" {
        n193 = Unbundle By Name(w560) -> ("main input"=w558:T4, "sub input"=w557:T4, "boolean high"=w553:sgl, "boolean low"=w552:sgl)
        n194 = Index Array(array=w559, index #1=w558, index #2=w557) -> (element #1=w556:bool, element #2=w555:bool)
        n195 = And(x=w556, y=w555) -> (x .and. y?=w554:bool)
        n196 = Select(t=w553, s=w554, f=w552) -> (s? t:f=w551:sgl)
      }
      frame "OR GATE" {
        n197 = Unbundle By Name(w564) -> ("main input"=w571:T4, "sub input"=w570:T4, "boolean high"=w566:sgl, "boolean low"=w565:sgl)
        n198 = Index Array(array=w563, index #1=w571, index #2=w570) -> (element #1=w569:bool, element #2=w568:bool)
        n199 = Or(x=w569, y=w568) -> (x .or. y?=w567:bool)
        n200 = Select(t=w566, s=w567, f=w565) -> (s? t:f=w562:sgl)
      }
      frame "ITERATION" {
        n201 = Unbundle By Name(w588) -> ("scan end"=w575:sgl, "scan begin"=w576:sgl, "scan step"=w585:sgl, "main input"=w586:T4)
        n202 = Add(x=w578, y=w585) -> (x+y=w583:sgl)
        n203 = Not(x=w582) -> (.not. x?=w581:bool)
        n204 = Index Array(array=w587, index=w586) -> (element=w580:bool)
        n205 = Greater?(x=w583, y=w575) -> (0:w584:bool)
        n206 = And(x=w580, y=w581) -> (x .and. y?=w579:bool)
        n207 = Select(t=w576, s=w584, f=w583) -> (s? t:f=w577:sgl)
        n208 = Select(t=w577, s=w579, f=w578) -> (s? t:f=w574:sgl)
        n209 = Select(t=w576, s=w572, f=w574) -> (s? t:f=w573:sgl)
      }
    }
    n210 = case shown="\"ITERATION\"" w73 {
      tunnel: [sgl 0.0 w493 w502 w513 w524] -> w65
      tunnel: w33 -> [_ w500 w510 w514 w538]
      tunnel: "Channel9" -> [_ w499 w511 w515 w539]
      tunnel: w49 -> [_ _ _ _ w529]
      tunnel: [FALSE ("Mod2/DIO31") FALSE ("Mod2/DIO31") FALSE ("Mod2/DIO31") FALSE ("Mod2/DIO31") w531] -> w64
      tunnel: w48 -> [_ _ _ _ w533]
      tunnel: w7 -> [_ _ _ _ w523]
      frame "OFF", Default {
      }
      frame "SWITCH" {
        n211 = Unbundle By Name(w499) -> ("boolean high"=w495:sgl, "boolean low"=w496:sgl, "main input"=w498:T4)
        n212 = Index Array(array=w500, index=w498) -> (element=w497:bool)
        n213 = Select(t=w495, s=w497, f=w496) -> (s? t:f=w493:sgl)
      }
      frame "AND GATE" {
        n214 = Unbundle By Name(w511) -> ("main input"=w509:T4, "sub input"=w508:T4, "boolean high"=w504:sgl, "boolean low"=w503:sgl)
        n215 = Index Array(array=w510, index #1=w509, index #2=w508) -> (element #1=w507:bool, element #2=w506:bool)
        n216 = And(x=w507, y=w506) -> (x .and. y?=w505:bool)
        n217 = Select(t=w504, s=w505, f=w503) -> (s? t:f=w502:sgl)
      }
      frame "OR GATE" {
        n218 = Unbundle By Name(w515) -> ("main input"=w522:T4, "sub input"=w521:T4, "boolean high"=w517:sgl, "boolean low"=w516:sgl)
        n219 = Index Array(array=w514, index #1=w522, index #2=w521) -> (element #1=w520:bool, element #2=w519:bool)
        n220 = Or(x=w520, y=w519) -> (x .or. y?=w518:bool)
        n221 = Select(t=w517, s=w518, f=w516) -> (s? t:f=w513:sgl)
      }
      frame "ITERATION" {
        n222 = Unbundle By Name(w539) -> ("scan end"=w526:sgl, "scan begin"=w527:sgl, "scan step"=w536:sgl, "main input"=w537:T4)
        n223 = Add(x=w529, y=w536) -> (x+y=w534:sgl)
        n224 = Not(x=w533) -> (.not. x?=w532:bool)
        n225 = Index Array(array=w538, index=w537) -> (element=w531:bool)
        n226 = Greater?(x=w534, y=w526) -> (0:w535:bool)
        n227 = And(x=w531, y=w532) -> (x .and. y?=w530:bool)
        n228 = Select(t=w527, s=w535, f=w534) -> (s? t:f=w528:sgl)
        n229 = Select(t=w528, s=w530, f=w529) -> (s? t:f=w525:sgl)
        n230 = Select(t=w527, s=w523, f=w525) -> (s? t:f=w524:sgl)
      }
    }
    n231 = case shown="\"ITERATION\"" w71 {
      tunnel: [sgl 0.0 w395 w404 w415 w426] -> w61
      tunnel: w33 -> [_ w402 w412 w416 w440]
      tunnel: "Channel6" -> [_ w401 w413 w417 w441]
      tunnel: w45 -> [_ _ _ _ w431]
      tunnel: [FALSE ("Mod2/DIO31") FALSE ("Mod2/DIO31") FALSE ("Mod2/DIO31") FALSE ("Mod2/DIO31") w433] -> w60
      tunnel: w44 -> [_ _ _ _ w435]
      tunnel: w10 -> [_ _ _ _ w425]
      frame "OFF", Default {
      }
      frame "SWITCH" {
        n232 = Unbundle By Name(w401) -> ("boolean high"=w397:sgl, "boolean low"=w398:sgl, "main input"=w400:T4)
        n233 = Index Array(array=w402, index=w400) -> (element=w399:bool)
        n234 = Select(t=w397, s=w399, f=w398) -> (s? t:f=w395:sgl)
      }
      frame "AND GATE" {
        n235 = Unbundle By Name(w413) -> ("main input"=w411:T4, "sub input"=w410:T4, "boolean high"=w406:sgl, "boolean low"=w405:sgl)
        n236 = Index Array(array=w412, index #1=w411, index #2=w410) -> (element #1=w409:bool, element #2=w408:bool)
        n237 = And(x=w409, y=w408) -> (x .and. y?=w407:bool)
        n238 = Select(t=w406, s=w407, f=w405) -> (s? t:f=w404:sgl)
      }
      frame "OR GATE" {
        n239 = Unbundle By Name(w417) -> ("main input"=w424:T4, "sub input"=w423:T4, "boolean high"=w419:sgl, "boolean low"=w418:sgl)
        n240 = Index Array(array=w416, index #1=w424, index #2=w423) -> (element #1=w422:bool, element #2=w421:bool)
        n241 = Or(x=w422, y=w421) -> (x .or. y?=w420:bool)
        n242 = Select(t=w419, s=w420, f=w418) -> (s? t:f=w415:sgl)
      }
      frame "ITERATION" {
        n243 = Unbundle By Name(w441) -> ("scan end"=w428:sgl, "scan begin"=w429:sgl, "scan step"=w438:sgl, "main input"=w439:T4)
        n244 = Add(x=w431, y=w438) -> (x+y=w436:sgl)
        n245 = Not(x=w435) -> (.not. x?=w434:bool)
        n246 = Index Array(array=w440, index=w439) -> (element=w433:bool)
        n247 = Greater?(x=w436, y=w428) -> (0:w437:bool)
        n248 = And(x=w433, y=w434) -> (x .and. y?=w432:bool)
        n249 = Select(t=w429, s=w437, f=w436) -> (s? t:f=w430:sgl)
        n250 = Select(t=w430, s=w432, f=w431) -> (s? t:f=w427:sgl)
        n251 = Select(t=w429, s=w425, f=w427) -> (s? t:f=w426:sgl)
      }
    }
    n252 = case shown="\"ITERATION\"" w68 {
      tunnel: [sgl 0.0 w248 w257 w268 w279] -> w55
      tunnel: w33 -> [_ w255 w265 w269 w293]
      tunnel: "Channel13" -> [_ w254 w266 w270 w294]
      tunnel: w39 -> [_ _ _ _ w284]
      tunnel: [FALSE ("Mod2/DIO31") FALSE ("Mod2/DIO31") FALSE ("Mod2/DIO31") FALSE ("Mod2/DIO31") w286] -> w54
      tunnel: w38 -> [_ _ _ _ w288]
      tunnel: w3 -> [_ _ _ _ w278]
      frame "OFF", Default {
      }
      frame "SWITCH" {
        n253 = Unbundle By Name(w254) -> ("boolean high"=w250:sgl, "boolean low"=w251:sgl, "main input"=w253:T4)
        n254 = Index Array(array=w255, index=w253) -> (element=w252:bool)
        n255 = Select(t=w250, s=w252, f=w251) -> (s? t:f=w248:sgl)
      }
      frame "AND GATE" {
        n256 = Unbundle By Name(w266) -> ("main input"=w264:T4, "sub input"=w263:T4, "boolean high"=w259:sgl, "boolean low"=w258:sgl)
        n257 = Index Array(array=w265, index #1=w264, index #2=w263) -> (element #1=w262:bool, element #2=w261:bool)
        n258 = And(x=w262, y=w261) -> (x .and. y?=w260:bool)
        n259 = Select(t=w259, s=w260, f=w258) -> (s? t:f=w257:sgl)
      }
      frame "OR GATE" {
        n260 = Unbundle By Name(w270) -> ("main input"=w277:T4, "sub input"=w276:T4, "boolean high"=w272:sgl, "boolean low"=w271:sgl)
        n261 = Index Array(array=w269, index #1=w277, index #2=w276) -> (element #1=w275:bool, element #2=w274:bool)
        n262 = Or(x=w275, y=w274) -> (x .or. y?=w273:bool)
        n263 = Select(t=w272, s=w273, f=w271) -> (s? t:f=w268:sgl)
      }
      frame "ITERATION" {
        n264 = Unbundle By Name(w294) -> ("scan end"=w281:sgl, "scan begin"=w282:sgl, "scan step"=w291:sgl, "main input"=w292:T4)
        n265 = Add(x=w284, y=w291) -> (x+y=w289:sgl)
        n266 = Not(x=w288) -> (.not. x?=w287:bool)
        n267 = Index Array(array=w293, index=w292) -> (element=w286:bool)
        n268 = Greater?(x=w289, y=w281) -> (0:w290:bool)
        n269 = And(x=w286, y=w287) -> (x .and. y?=w285:bool)
        n270 = Select(t=w282, s=w290, f=w289) -> (s? t:f=w283:sgl)
        n271 = Select(t=w283, s=w285, f=w284) -> (s? t:f=w280:sgl)
        n272 = Select(t=w282, s=w278, f=w280) -> (s? t:f=w279:sgl)
      }
    }
    n273 = case shown="\"ITERATION\"" w69 {
      tunnel: [sgl 0.0 w297 w306 w317 w328] -> w57
      tunnel: w33 -> [_ w304 w314 w318 w342]
      tunnel: "Channel12" -> [_ w303 w315 w319 w343]
      tunnel: w41 -> [_ _ _ _ w333]
      tunnel: [FALSE ("Mod2/DIO31") FALSE ("Mod2/DIO31") FALSE ("Mod2/DIO31") FALSE ("Mod2/DIO31") w335] -> w56
      tunnel: w40 -> [_ _ _ _ w337]
      tunnel: w4 -> [_ _ _ _ w327]
      frame "OFF", Default {
      }
      frame "SWITCH" {
        n274 = Unbundle By Name(w303) -> ("boolean high"=w299:sgl, "boolean low"=w300:sgl, "main input"=w302:T4)
        n275 = Index Array(array=w304, index=w302) -> (element=w301:bool)
        n276 = Select(t=w299, s=w301, f=w300) -> (s? t:f=w297:sgl)
      }
      frame "AND GATE" {
        n277 = Unbundle By Name(w315) -> ("main input"=w313:T4, "sub input"=w312:T4, "boolean high"=w308:sgl, "boolean low"=w307:sgl)
        n278 = Index Array(array=w314, index #1=w313, index #2=w312) -> (element #1=w311:bool, element #2=w310:bool)
        n279 = And(x=w311, y=w310) -> (x .and. y?=w309:bool)
        n280 = Select(t=w308, s=w309, f=w307) -> (s? t:f=w306:sgl)
      }
      frame "OR GATE" {
        n281 = Unbundle By Name(w319) -> ("main input"=w326:T4, "sub input"=w325:T4, "boolean high"=w321:sgl, "boolean low"=w320:sgl)
        n282 = Index Array(array=w318, index #1=w326, index #2=w325) -> (element #1=w324:bool, element #2=w323:bool)
        n283 = Or(x=w324, y=w323) -> (x .or. y?=w322:bool)
        n284 = Select(t=w321, s=w322, f=w320) -> (s? t:f=w317:sgl)
      }
      frame "ITERATION" {
        n285 = Unbundle By Name(w343) -> ("scan end"=w330:sgl, "scan begin"=w331:sgl, "scan step"=w340:sgl, "main input"=w341:T4)
        n286 = Add(x=w333, y=w340) -> (x+y=w338:sgl)
        n287 = Not(x=w337) -> (.not. x?=w336:bool)
        n288 = Index Array(array=w342, index=w341) -> (element=w335:bool)
        n289 = Greater?(x=w338, y=w330) -> (0:w339:bool)
        n290 = And(x=w335, y=w336) -> (x .and. y?=w334:bool)
        n291 = Select(t=w331, s=w339, f=w338) -> (s? t:f=w332:sgl)
        n292 = Select(t=w332, s=w334, f=w333) -> (s? t:f=w329:sgl)
        n293 = Select(t=w331, s=w327, f=w329) -> (s? t:f=w328:sgl)
      }
    }
    n294 = case shown="\"ITERATION\"" w67 {
      tunnel: [sgl 0.0 w199 w208 w219 w230] -> w53
      tunnel: w33 -> [_ w206 w216 w220 w244]
      tunnel: "Channel14" -> [_ w205 w217 w221 w245]
      tunnel: w37 -> [_ _ _ _ w235]
      tunnel: [FALSE ("Mod2/DIO31") FALSE ("Mod2/DIO31") FALSE ("Mod2/DIO31") FALSE ("Mod2/DIO31") w237] -> w52
      tunnel: w36 -> [_ _ _ _ w239]
      tunnel: w2 -> [_ _ _ _ w229]
      frame "OFF", Default {
      }
      frame "SWITCH" {
        n295 = Unbundle By Name(w205) -> ("boolean high"=w201:sgl, "boolean low"=w202:sgl, "main input"=w204:T4)
        n296 = Index Array(array=w206, index=w204) -> (element=w203:bool)
        n297 = Select(t=w201, s=w203, f=w202) -> (s? t:f=w199:sgl)
      }
      frame "AND GATE" {
        n298 = Unbundle By Name(w217) -> ("main input"=w215:T4, "sub input"=w214:T4, "boolean high"=w210:sgl, "boolean low"=w209:sgl)
        n299 = Index Array(array=w216, index #1=w215, index #2=w214) -> (element #1=w213:bool, element #2=w212:bool)
        n300 = And(x=w213, y=w212) -> (x .and. y?=w211:bool)
        n301 = Select(t=w210, s=w211, f=w209) -> (s? t:f=w208:sgl)
      }
      frame "OR GATE" {
        n302 = Unbundle By Name(w221) -> ("main input"=w228:T4, "sub input"=w227:T4, "boolean high"=w223:sgl, "boolean low"=w222:sgl)
        n303 = Index Array(array=w220, index #1=w228, index #2=w227) -> (element #1=w226:bool, element #2=w225:bool)
        n304 = Or(x=w226, y=w225) -> (x .or. y?=w224:bool)
        n305 = Select(t=w223, s=w224, f=w222) -> (s? t:f=w219:sgl)
      }
      frame "ITERATION" {
        n306 = Unbundle By Name(w245) -> ("scan end"=w232:sgl, "scan begin"=w233:sgl, "scan step"=w242:sgl, "main input"=w243:T4)
        n307 = Add(x=w235, y=w242) -> (x+y=w240:sgl)
        n308 = Not(x=w239) -> (.not. x?=w238:bool)
        n309 = Index Array(array=w244, index=w243) -> (element=w237:bool)
        n310 = Greater?(x=w240, y=w232) -> (0:w241:bool)
        n311 = And(x=w237, y=w238) -> (x .and. y?=w236:bool)
        n312 = Select(t=w233, s=w241, f=w240) -> (s? t:f=w234:sgl)
        n313 = Select(t=w234, s=w236, f=w235) -> (s? t:f=w231:sgl)
        n314 = Select(t=w233, s=w229, f=w231) -> (s? t:f=w230:sgl)
      }
    }
    n315 = case shown="\"ITERATION\"" w66 {
      tunnel: [sgl 0.0 w150 w159 w170 w181] -> w51
      tunnel: w33 -> [_ w157 w167 w171 w195]
      tunnel: "Channel15" -> [_ w156 w168 w172 w196]
      tunnel: w35 -> [_ _ _ _ w186]
      tunnel: [FALSE ("Mod2/DIO31") FALSE ("Mod2/DIO31") FALSE ("Mod2/DIO31") FALSE ("Mod2/DIO31") w188] -> w50
      tunnel: w34 -> [_ _ _ _ w190]
      tunnel: w1 -> [_ _ _ _ w180]
      frame "OFF", Default {
      }
      frame "SWITCH" {
        n316 = Unbundle By Name(w156) -> ("boolean high"=w152:sgl, "boolean low"=w153:sgl, "main input"=w155:T4)
        n317 = Index Array(array=w157, index=w155) -> (element=w154:bool)
        n318 = Select(t=w152, s=w154, f=w153) -> (s? t:f=w150:sgl)
      }
      frame "AND GATE" {
        n319 = Unbundle By Name(w168) -> ("main input"=w166:T4, "sub input"=w165:T4, "boolean high"=w161:sgl, "boolean low"=w160:sgl)
        n320 = Index Array(array=w167, index #1=w166, index #2=w165) -> (element #1=w164:bool, element #2=w163:bool)
        n321 = And(x=w164, y=w163) -> (x .and. y?=w162:bool)
        n322 = Select(t=w161, s=w162, f=w160) -> (s? t:f=w159:sgl)
      }
      frame "OR GATE" {
        n323 = Unbundle By Name(w172) -> ("main input"=w179:T4, "sub input"=w178:T4, "boolean high"=w174:sgl, "boolean low"=w173:sgl)
        n324 = Index Array(array=w171, index #1=w179, index #2=w178) -> (element #1=w177:bool, element #2=w176:bool)
        n325 = Or(x=w177, y=w176) -> (x .or. y?=w175:bool)
        n326 = Select(t=w174, s=w175, f=w173) -> (s? t:f=w170:sgl)
      }
      frame "ITERATION" {
        n327 = Unbundle By Name(w196) -> ("scan end"=w183:sgl, "scan begin"=w184:sgl, "scan step"=w193:sgl, "main input"=w194:T4)
        n328 = Add(x=w186, y=w193) -> (x+y=w191:sgl)
        n329 = Not(x=w190) -> (.not. x?=w189:bool)
        n330 = Index Array(array=w195, index=w194) -> (element=w188:bool)
        n331 = Greater?(x=w191, y=w183) -> (0:w192:bool)
        n332 = And(x=w188, y=w189) -> (x .and. y?=w187:bool)
        n333 = Select(t=w184, s=w192, f=w191) -> (s? t:f=w185:sgl)
        n334 = Select(t=w185, s=w187, f=w186) -> (s? t:f=w182:sgl)
        n335 = Select(t=w184, s=w180, f=w182) -> (s? t:f=w181:sgl)
      }
    }
    n336 = case shown="\"ITERATION\"" w70 {
      tunnel: [sgl 0.0 w346 w355 w366 w377] -> w59
      tunnel: w33 -> [_ w353 w363 w367 w391]
      tunnel: "Channel7" -> [_ w352 w364 w368 w392]
      tunnel: w43 -> [_ _ _ _ w382]
      tunnel: [FALSE ("Mod2/DIO31") FALSE ("Mod2/DIO31") FALSE ("Mod2/DIO31") FALSE ("Mod2/DIO31") w384] -> w58
      tunnel: w42 -> [_ _ _ _ w386]
      tunnel: w9 -> [_ _ _ _ w376]
      frame "OFF", Default {
      }
      frame "SWITCH" {
        n337 = Unbundle By Name(w352) -> ("boolean high"=w348:sgl, "boolean low"=w349:sgl, "main input"=w351:T4)
        n338 = Index Array(array=w353, index=w351) -> (element=w350:bool)
        n339 = Select(t=w348, s=w350, f=w349) -> (s? t:f=w346:sgl)
      }
      frame "AND GATE" {
        n340 = Unbundle By Name(w364) -> ("main input"=w362:T4, "sub input"=w361:T4, "boolean high"=w357:sgl, "boolean low"=w356:sgl)
        n341 = Index Array(array=w363, index #1=w362, index #2=w361) -> (element #1=w360:bool, element #2=w359:bool)
        n342 = And(x=w360, y=w359) -> (x .and. y?=w358:bool)
        n343 = Select(t=w357, s=w358, f=w356) -> (s? t:f=w355:sgl)
      }
      frame "OR GATE" {
        n344 = Unbundle By Name(w368) -> ("main input"=w375:T4, "sub input"=w374:T4, "boolean high"=w370:sgl, "boolean low"=w369:sgl)
        n345 = Index Array(array=w367, index #1=w375, index #2=w374) -> (element #1=w373:bool, element #2=w372:bool)
        n346 = Or(x=w373, y=w372) -> (x .or. y?=w371:bool)
        n347 = Select(t=w370, s=w371, f=w369) -> (s? t:f=w366:sgl)
      }
      frame "ITERATION" {
        n348 = Unbundle By Name(w392) -> ("scan end"=w379:sgl, "scan begin"=w380:sgl, "scan step"=w389:sgl, "main input"=w390:T4)
        n349 = Add(x=w382, y=w389) -> (x+y=w387:sgl)
        n350 = Not(x=w386) -> (.not. x?=w385:bool)
        n351 = Index Array(array=w391, index=w390) -> (element=w384:bool)
        n352 = Greater?(x=w387, y=w379) -> (0:w388:bool)
        n353 = And(x=w384, y=w385) -> (x .and. y?=w383:bool)
        n354 = Select(t=w380, s=w388, f=w387) -> (s? t:f=w381:sgl)
        n355 = Select(t=w381, s=w383, f=w382) -> (s? t:f=w378:sgl)
        n356 = Select(t=w380, s=w376, f=w378) -> (s? t:f=w377:sgl)
      }
    }
    n357 = xnode "FPGA I/O Node"("Mod4/AO0"=w113) -> ()  [unwired: 1 in, 1 out]
    n358 = xnode "FPGA I/O Node"("Mod4/AO1"=w107) -> ()  [unwired: 1 in, 1 out]
    n359 = xnode "FPGA I/O Node"("Mod4/AO2"=w99) -> ()  [unwired: 1 in, 1 out]
    n360 = xnode "FPGA I/O Node"("Mod4/AO3"=w101) -> ()  [unwired: 1 in, 1 out]
    n361 = xnode "FPGA I/O Node"("Mod4/AO4"=w89) -> ()  [unwired: 1 in, 1 out]
    n362 = xnode "FPGA I/O Node"("Mod4/AO5"=w87) -> ()  [unwired: 1 in, 1 out]
    n363 = xnode "FPGA I/O Node"("Mod4/AO11"=w85) -> ()  [unwired: 1 in, 1 out]
    n364 = xnode "FPGA I/O Node"("Mod4/AO10"=w63) -> ()  [unwired: 1 in, 1 out]
    n365 = xnode "FPGA I/O Node"("Mod4/AO8"=w83) -> ()  [unwired: 1 in, 1 out]
    n366 = xnode "FPGA I/O Node"("Mod4/AO9"=w65) -> ()  [unwired: 1 in, 1 out]
    n367 = xnode "FPGA I/O Node"("Mod4/AO6"=w61) -> ()  [unwired: 1 in, 1 out]
    n368 = xnode "FPGA I/O Node"("Mod4/AO13"=w55) -> ()  [unwired: 1 in, 1 out]
    n369 = xnode "FPGA I/O Node"("Mod4/AO12"=w57) -> ()  [unwired: 1 in, 1 out]
    n370 = xnode "FPGA I/O Node"("Mod4/AO14"=w53) -> ()  [unwired: 1 in, 1 out]
    n371 = xnode "FPGA I/O Node"("Mod4/AO15"=w51) -> ()  [unwired: 1 in, 1 out]
    n372 = xnode "FPGA I/O Node"("Mod4/AO7"=w59) -> ()  [unwired: 1 in, 1 out]
  }
